vi "Set User Event.vi"(11 "userEvent":u32) -> (2 "function return":u32, 3 "userEvent out":u32)   [LabVIEW 2018, in "AndorSDK.lvlib"]
doc: "EXPNETTYPE unsigned int WINAPI SetUserEvent(HANDLE userEvent);"
uses:
  AndorSDK.lvlib
  ATMCD32D.dll
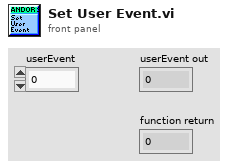
[diagram p1: front panel]
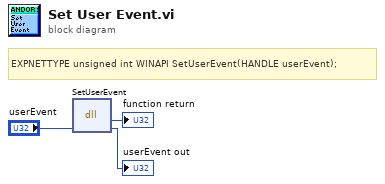
[diagram p0: block diagram]
diagram:
  # "EXPNETTYPE unsigned int WINAPI SetUserEvent(HANDLE userEvent);"
  n1 = dll-call lib="PTH2babs E\nPersönliches02 - Arbeit03-HiwijobsLabviewCodelibANDOR\tAndor SDK\nATMCD32D.*" fn="SetUserEvent"("userEvent"="userEvent") -> (→"function return":u32, "userEvent"=→"userEvent out":u32)  [unwired: 3 in, 2 out]
